vi "Task1.vi"() -> ()   [LabVIEW 2021]
uses:
  <vilib>/myRIO/Common/Instrument Driver Framework/myRIO v1.0/DIO/vis/myRIO v1.0 Close DIO.vi
  <vilib>/myRIO/Common/Instrument Driver Framework/myRIO v1.0/DIO/vis/myRIO v1.0 Unreserve DIO.vi
  <vilib>/myRIO/Common/Instrument Driver Framework/myRIO v1.0/DIO/vis/myRIO v1.0 Build MUX Configuration DIO.vi
  <vilib>/myRIO/Common/Instrument Driver Framework/myRIO v1.0/Resource Manager/vis/myRIO v1.0 Unreserve Channel List.vi
  <vilib>/myRIO/Common/Instrument Driver Framework/myRIO v1.0/Resource Manager/vis/myRIO v1.0 Create Configuration List.vi
  <vilib>/myRIO/Common/Instrument Driver Framework/myRIO v1.0/Resource Manager/vis/myRIO v1.0 Unreserve Channel.vi
  <vilib>/myRIO/Common/Instrument Driver Framework/myRIO v1.0/Resource Manager/vis/myRIO v1.0 Build Mutex Name.vi
  <vilib>/Utility/error.llb/Error Cluster From Error Code.vi
  <vilib>/myRIO/Common/Instrument Driver Framework/myRIO v1.0/DIO/vis/myRIO v1.0 Write DIO.vi
  <vilib>/myRIO/Common/Instrument Driver Framework/myRIO v1.0/DIO/vis/myRIO v1.0 Shutdown DIO.vi
  <vilib>/myRIO/Common/Instrument Driver Framework/myRIO v1.0/Resource Manager/vis/myRIO v1.0 Configure IO.vi
  <vilib>/myRIO/Common/Instrument Driver Framework/Utilities/vis/Configuration Manager.vi
  <vilib>/myRIO/Common/Instrument Driver Framework/Utilities/vis/IO Manager.vi
  <vilib>/myRIO/Common/Instrument Driver Framework/myRIO v1.0/myRIO v1.0 Close.vi
  <vilib>/myRIO/Instrument Drivers/Onboard IO/DIO/DIO.lvlib
panel:
  out "floor(x/y)":i32
  in  "stop":bool
  in  "RPM":dbl(slide) scale=0.1..10.0
  out "Visualize":bool[](array[boolean])
  in  "Full Step":bool
  in  "Direction":enum32{"CW", "CCW"}(radio)
  # "Half Step"
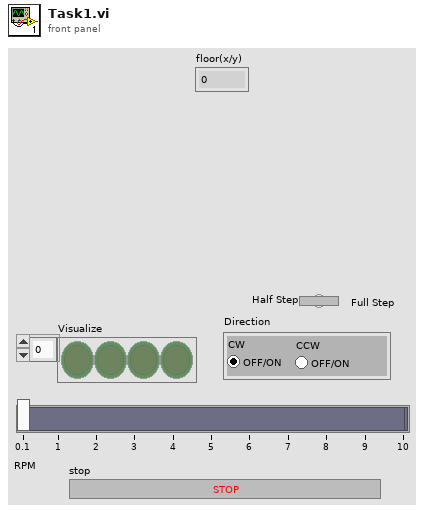
[diagram p1: front panel]
types:
  T1 = typedef "DIO.lvlib/DIO Reference.ctl" = cluster{"myRIO Reference":T2, "DIO Channels List":T6}
  T2 = typedef "myRIO Generic Hardware Reference.ctl" = cluster{"myRIO Model":T3, "myRIO Hardware Reference":T4}
  T3 = typedef "Hardware Version Enum.ctl" = enum16{"Unknown", "myRIO-1900", "myRIO-1950", "roboRIO", "NI ELVIS RIO CM", "ELVIS III"}
  T4 = typedef "myRIO v1.0 Reference.ctl" = cluster{"Generic FPGA Reference":T5, "Allow multiple opens":bool}
  T5 = typedef "Generic FPGA Reference.ctl" = refnum<k20>
  T6 = typedef "DIO Channels List.ctl" = T7[]
  T7 = typedef "DIO Channels Enum.ctl" = enum16{"Not Connected", "C/DIO0", "C/DIO1", "C/DIO2", "C/DIO3", "C/DIO4", "C/DIO5", "C/DIO6", "C/DIO7", "A/DIO0", "A/DIO1", "A/DIO2", "A/DIO3", "A/DIO4", "A/DIO5", "A/DIO6", "A/DIO7", "A/DIO8", "A/DIO9", "A/DIO10", "A/DIO11", "A/DIO12", "A/DIO13", "A/DIO14", "A/DIO15", "A/DIO16", "A/DIO17", "A/DIO18", "A/DIO19", "B/DIO0", "B/DIO1", "B/DIO2", "B/DIO3", "B/DIO4", "B/DIO5", "B/DIO6", "B/DIO7", "B/DIO8", "B/DIO9", "B/DIO10", "B/DIO11", "B/DIO12", "B/DIO13", "B/DIO14", "B/DIO15", "B/DIO16", "B/DIO17", "B/DIO18", "B/DIO19", "LED0", "LED1", "LED2", "LED3", "Button0", "DIO/DIO0", "DIO/DIO1", "DIO/DIO2", "DIO/DIO3", "DIO/DIO4", "DIO/DIO5", "DIO/DIO6", "DIO/DIO7", "DIO/DIO8", "DIO/DIO9", "SPI/CS0", "SPI/CS1", "SPI/CS2", "SPI/CS3", "LED RADIO (Green)", "LED RADIO (Red)", "LED COMM (Green)", "LED COMM (Red)", "LED MODE (Green)", "LED MODE (Red)"}
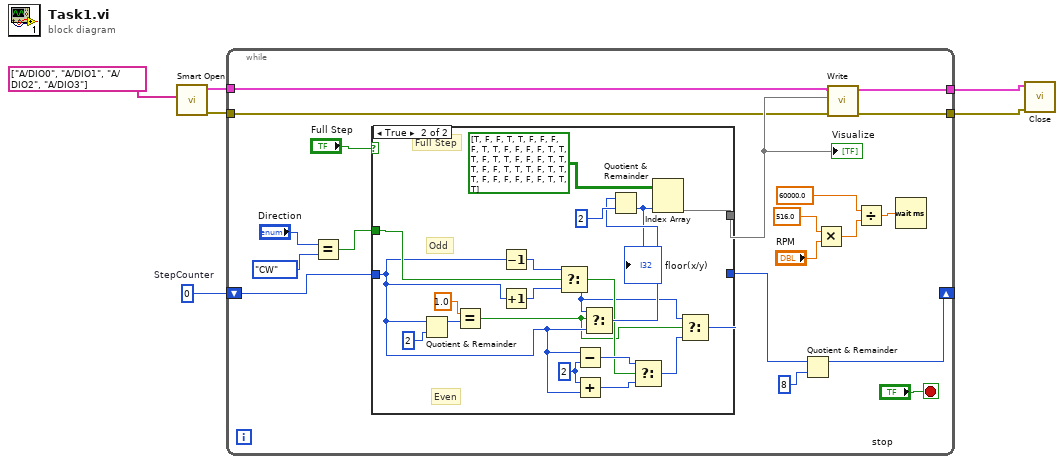
[diagram p0: block diagram]
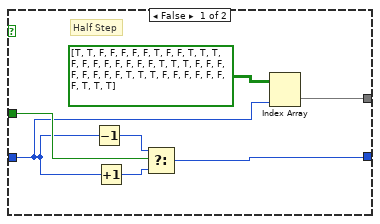
[diagram p2: hidden frame]
diagram:
  w6 = 0  # StepCounter
  n1 = call <vilib>:"Smart Open.vi"("Channel Names"=tag[] ["A/DIO0", "A/DIO1", "A/DIO2", "A/DIO3"]) -> ("error out"=w3:errorcluster, "DIO Ref Out"=w4:T1)  [unwired: 9 in]
  n2 = while {
    shift-right: [w20] -> _
    shift-left: w6 -> [w23]
    tunnel: w3 -> [w9]
    tunnel: w4 -> [w11]
    tunnel: [w8] -> w2
    tunnel: [w7] -> w1
    stop <- "stop" stop-if-true
    n3 = Equal?(x="Direction", y=enum32{"CW", "CCW"}."CW") -> (x = y?=w17:bool)
    n4 = case shown="True" "Full Step" {
      tunnel: w23 -> [w26 w37]
      tunnel: [w28 w33] -> w22
      tunnel: w17 -> [w32 w39]
      tunnel: [w31 w41] -> w10
      frame False {
        # "Half Step"
        n5 = Decrement(x=w26) -> (x-1=w30:i32)
        n6 = Increment(x=w26) -> (x+1=w29:i32)
        n7 = Select(t=w30, s=w32, f=w29) -> (s? t:f=w28:i32)
        n8 = Index Array(array=bool[][] [[TRUE, TRUE, FALSE, FALSE, FALSE, FALSE, FALSE, TRUE, FALSE], [FALSE, TRUE, TRUE, TRUE, FALSE, FALSE, FALSE, FALSE, FALSE], [FALSE, FALSE, FALSE, TRUE, TRUE, TRUE, FALSE, FALSE, FALSE], [FALSE, FALSE, FALSE, FALSE, FALSE, TRUE, TRUE, TRUE, FALSE], [FALSE, FALSE, FALSE, FALSE, FALSE, FALSE, TRUE, TRUE, TRUE]], index (col)=w26) -> (element=w31:bool[])  [unwired: 1 in]
      }
      frame True {
        w51 = 2 ("y")
        # "Odd"
        # "Even"
        # "Full Step"
        n9 = Quotient & Remainder(x=w37, y=2) -> (x-y*floor(x/y)=w47:i32)  [unwired: 1 out]
        n10 = Equal?(x=1.0, y=w47) -> (x = y?=w36:bool)
        n11 = Decrement(x=w37) -> (x-1=w46:i32)
        n12 = Increment(x=w37) -> (x+1=w45:i32)
        n13 = Select(t=w46, s=w39, f=w45) -> (s? t:f=w35:i32)
        n14 = Subtract(x=w37, y=w51) -> (x-y=w50:i32)
        n15 = Add(x=w51, y=w37) -> (x+y=w44:i32)
        n16 = Select(t=w35, s=w36, f=w37) -> (s? t:f=w40:i32)
        n17 = Quotient & Remainder(x=w40, y=2) -> (floor(x/y)=w38:i32)  [unwired: 1 out]
        "floor(x/y)" <- w38
        n18 = Select(t=w50, s=w39, f=w44) -> (s? t:f=w34:i32)
        n19 = Index Array(array=bool[][] [[TRUE, FALSE, FALSE, TRUE, TRUE, FALSE, FALSE, FALSE, FALSE], [TRUE, TRUE, FALSE, FALSE, FALSE, FALSE, TRUE, TRUE, TRUE], [FALSE, TRUE, TRUE, FALSE, FALSE, FALSE, TRUE, TRUE, TRUE], [FALSE, FALSE, TRUE, TRUE, TRUE, FALSE, TRUE, TRUE, TRUE], [FALSE, FALSE, FALSE, FALSE, FALSE, FALSE, TRUE, TRUE, TRUE]], index (col)=w38) -> (element=w41:bool[])  [unwired: 1 in]
        n20 = Select(t=w35, s=w36, f=w34) -> (s? t:f=w33:i32)
      }
    }
    "Visualize" <- w10
    n21 = Quotient & Remainder(x=w22, y=8) -> (x-y*floor(x/y)=w20:i32)  [unwired: 1 out]
    n22 = Multiply(x=516.0 ("y"), y="RPM") -> (x*y=w15:dbl)
    n23 = call <vilib>:"Write.vi"("error in (no error)"=w9, "Values"=w10, "DIO Ref In"=w11) -> ("error out"=w7:errorcluster, "DIO Ref Out"=w8:T1)  [unwired: 6 in]
    n24 = Divide(x=60000.0 ("y"), y=w15) -> (x/y=w12:dbl)
    n25 = Wait (ms)(milliseconds to wait=w12) -> ()  [unwired: 1 out]
  }
  n26 = call <vilib>:"Close.vi"("error in (no error)"=w1, "DIO Ref In"=w2) -> ()  [unwired: 9 in, 1 out]
